vi "Resize and Position jpg.vi"(6 "New Height":i16=120, 8 "Pos y":i16=125, 9 "Pos x":i16=280, 10 "appended path":path, 11 "Picture In":picture) -> (3 "Picture Out":picture)   [LabVIEW 2014]
uses:
  <vilib>/picture/picture.llb/Draw True-Color Pixmap.vi
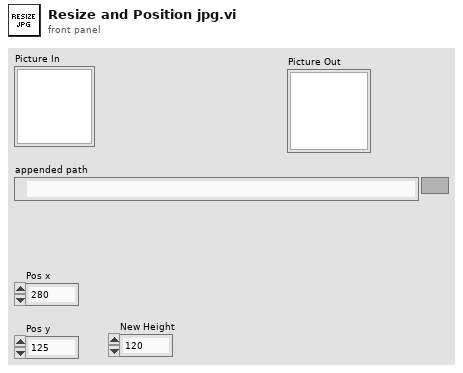
[diagram p1: front panel]
types:
  T1 = typedef "imagedata.ctl" = cluster{"image type":i32, "image depth":i32, "image":u8[], "mask":u8[], "colors":u32[], "Rectangle":cluster{"left":i16, "top":i16, "right":i16, "bottom":i16}}
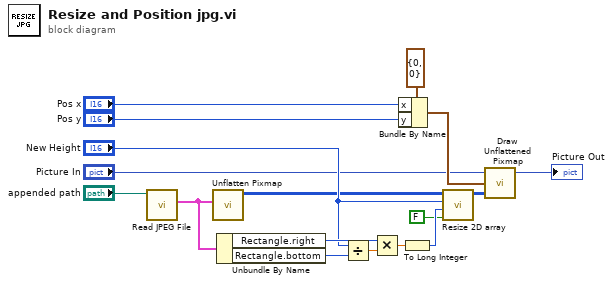
[diagram p0: block diagram]
diagram:
  n1 = call <vilib>:"Read JPEG File.vi"("path to JPEG file"="appended path") -> ("image data"=w8:T1)  [unwired: 8 in, 2 out]
  n2 = call <vilib>:"Unflatten Pixmap.vi"("image data"=w8) -> ("24-bit pixmap"=w1:u32[][])  [unwired: 4 in, 6 out]
  n3 = Unbundle By Name(w8) -> ("Rectangle.right"=w12:i16, "Rectangle.bottom"=w9:i16)
  n4 = Divide(x="New Height", y=w9) -> (x/y=w11:dbl)
  n5 = Multiply(x=w12, y=w11) -> (x*y=w13:dbl)
  n6 = Bundle By Name(cluster=cluster{"x":i16, "y":i16} {"x"=0, "y"=0} ("top left point(0, 0)"), "x"="Pos x", "y"="Pos y") -> (w6:cluster{"x":i16, "y":i16})
  n7 = To Long Integer(number=w13) -> (32bit integer=w14:i32)
  n8 = call "Resize 2D array.vi"("Maintain Aspect ratio? (T)"=FALSE, "New Width"=w14, "New Height"="New Height", "2D Array In"=w1) -> ("Resized Array"=w2:u32[][])  [unwired: 3 in]
  n9 = call-poly <vilib>:"Draw Unflattened Pixmap.vi"("picture"="Picture In", "top left point(0, 0)"=w6, "data (RGB format)"=w2) -> ("new picture"=→"Picture Out":picture)  [unwired: 6 in]
